vi "MapDestinationToSourcevi.vi"(2 "String":string) -> (6 "Dest > Source":T1(c390))   [LabVIEW 2022 SP3]
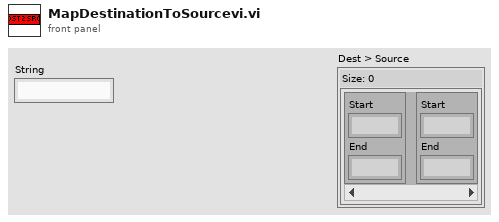
[diagram p1: front panel]
types:
  T1 = map{cluster{"Start":u64, "End":u64}, cluster{"Start":u64, "End":u64}}
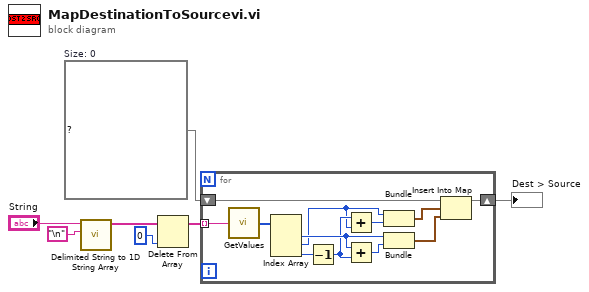
[diagram p0: block diagram]
diagram:
  w6 = T1 {}  # Size: 0
  n1 = call <vilib>:"Delimited String to 1D String Array.vi"("delimiter"="\n", "delimited string"="String") -> ("string array"=w4:string[])  [unwired: 9 in]
  n2 = Delete From Array(array=w4, index=0) -> (array with subset deleted=w7:string[])  [unwired: 1 in, 1 out]
  n3 = for {
    shift-right: [w16] -> w1
    shift-left: w6 -> [w17]
    tunnel: w7 -> [w19] mode=indexing
    n4 = call "GetValues.vi"("String"=w19) -> ("Values"=w18:u64[])  [unwired: 6 in]
    n5 = Index Array(array=w18) -> (element #1=w14:u64, element #2=w11:u64, element #3=w15:u64)  [unwired: 3 in]
    n6 = Decrement(x=w15) -> (x-1=w12:u64)
    n7 = Add(x=w12, y=w11) -> (x+y=w10:u64)
    n8 = Add(x=w14, y=w12) -> (x+y=w13:u64)
    n9 = Bundle(w11, w10) -> (w9:cluster{u64, u64})  [unwired: 1 in]
    n10 = Bundle(w14, w13) -> (w8:cluster{u64, u64})  [unwired: 1 in]
    n11 = Insert Into Map(map in=w17, key=w9, value=w8) -> (map out=w16:T1)  [unwired: 2 out]
  }
  "Dest > Source" <- w1
